vi "TEST - Initialize Array to Path Array.vi"(8 "error in (no error)":errorcluster) -> (0 "error out":errorcluster, 2 "Pass?":bool=TRUE)   [LabVIEW 2009]
doc: "This VI template can be used for the functional testing of VIs; this implementation includes handling for the testing of polymorphic VIs, and the polymorphic elements should be removed if not needed.\n\nCoded by Douglas A. Femec, January 24, 2006.\n\nCopyright (c) 2005-2006 MKS Instruments, Inc.\nAll rights reserved."
uses:
  TEST - Initialize Array from Array - Inputs.ctl
  tests/Polymorphizer+ Data Type.ctl
  TEST - Initialize Array from Array - Outputs.ctl
  Initialize Array from Array/Initialize 1D Array (Path) from 1D Array (EXT).vi
  Initialize Array from Array/Initialize 2D Array (Path) from 2D Array (EXT).vi
  Initialize Array from Array/Initialize 1D Array (Path) from 1D Array (DBL).vi
  Initialize Array from Array/Initialize 2D Array (Path) from 2D Array (DBL).vi
  Initialize Array from Array/Initialize 1D Array (Path) from 1D Array (SGL).vi
  Initialize Array from Array/Initialize 2D Array (Path) from 2D Array (SGL).vi
  Initialize Array from Array/Initialize 1D Array (Path) from 1D Array (I32).vi
  Initialize Array from Array/Initialize 2D Array (Path) from 2D Array (I32).vi
  Initialize Array from Array/Initialize 1D Array (Path) from 1D Array (I64).vi
  Initialize Array from Array/Initialize 2D Array (Path) from 2D Array (I64).vi
  Initialize Array from Array/Initialize 1D Array (Path) from 1D Array (U64).vi
  Initialize Array from Array/Initialize 1D Array (Path) from 1D Array (I16).vi
  Initialize Array from Array/Initialize 2D Array (Path) from 2D Array (I16).vi
  Initialize Array from Array/Initialize 1D Array (Path) from 1D Array (I8).vi
  Initialize Array from Array/Initialize 2D Array (Path) from 2D Array (I8).vi
  Initialize Array from Array/Initialize 1D Array (Path) from 1D Array (U32).vi
  Initialize Array from Array/Initialize 2D Array (Path) from 2D Array (U32).vi
  Initialize Array from Array/Initialize 1D Array (Path) from 1D Array (U16).vi
  Initialize Array from Array/Initialize 2D Array (Path) from 2D Array (U16).vi
  Initialize Array from Array/Initialize 1D Array (Path) from 1D Array (U8).vi
  Initialize Array from Array/Initialize 2D Array (Path) from 2D Array (U8).vi
  Initialize Array from Array/Initialize 1D Array (Path) from 1D Array (Boolean).vi
  Initialize Array from Array/Initialize 2D Array (Path) from 2D Array (Boolean).vi
  Initialize Array from Array/Initialize 1D Array (Path) from 1D Array (String).vi
  Initialize Array from Array/Initialize 2D Array (Path) from 2D Array (String).vi
  Initialize Array from Array/Initialize 1D Array (Path) from 1D Array (Path).vi
  Initialize Array from Array/Initialize 2D Array (Path) from 2D Array (Path).vi
  Initialize Array from Array/Initialize 1D Array (Path) from 1D Array (Variant).vi
  Initialize Array from Array/Initialize 2D Array (Path) from 2D Array (Variant).vi
panel:
  out "Generated Outputs":T1[][](array[typedef]) {"1D Array" format="%.2f"; "2D Array" format="%.2f"}
  in  "Expected Outputs":T1[](array[typedef])=[{"Description"="Expect empty arrays", "1D Array"=[], "2D Array"=[]}, {"Description"="Expect 1-element arrays", "1D Array"=[1.0], "2D Array"=[[1.0]]}, {"Description"="Expect 1-row arrays", "1D Array"=[1.0], "2D Array"=[[1.0, 1.0]]}, {"Description"="Expect 1-column arrays", "1D Array"=[1.0], "2D Array"=[[1.0], [1.0], [1.0], [1.0]]}, {"Description"="Expect 2-columns, 4-rows arrays", "1D Array"=[1.0, 1.0, 1.0, 1.0], "2D Array"=[[1.0, 1.0], [1.0, 1.0], [1.0, 1.0], [1.0, 1.0]]}] {"1D Array" format="%.2f"; "2D Array" format="%.2f"}
  in  "Inputs":T2[](array[typedef])=[{"Description"="Empty arrays", "Data Types to Test"=[enum."EXT", enum."DBL", enum."SGL", enum."I32", enum."I16", enum."I8", enum."U32", enum."U16", enum."U8", enum."Boolean", enum."String", enum."Path", enum."Variant", enum."I64", enum."U64"], "1D Array"=[], "2D Array"=[]}, {"Description"="1-Element arrays", "Data Types to Test"=[enum."EXT", enum."DBL", enum."SGL", enum."I32", enum."I16", enum."I8", enum."U32", enum."U16", enum."U8", enum."Boolean", enum."String", enum."Path", enum."Variant", enum."I64", enum."U64"], "1D Array"=[1.0], "2D Array"=[[1.0]]}, {"Description"="1-Row arrays", "Data Types to Test"=[enum."EXT", enum."DBL", enum."SGL", enum."I32", enum."I16", enum."I8", enum."U32", enum."U16", enum."U8", enum."Boolean", enum."String", enum."Path", enum."Variant", enum."I64", enum."U64"], "1D Array"=[1.0], "2D Array"=[[1.0, 1.0]]}, {"Description"="1-Column arrays", "Data Types to Test"=[enum."EXT", enum."DBL", enum."SGL", enum."I32", enum."I16", enum."I8", enum."U32", enum."U16", enum."U8", enum."Boolean", enum."String", enum."Path", enum."Variant", enum."I64", enum."U64"], "1D Array"=[1.0], "2D Array"=[[1.0], [1.0], [1.0], [1.0]]}, {"Description"="2-Columns, 4-rows arrays", "Data Types to Test"=[enum."EXT", enum."DBL", enum."SGL", enum."I32", enum."I16", enum."I8", enum."U32", enum."U16", enum."U8", enum."Boolean", enum."String", enum."Path", enum."Variant", enum."I64", enum."U64"], "1D Array"=[1.0, 1.0, 1.0, 1.0], "2D Array"=[[1.0, 1.0], [1.0, 1.0], [1.0, 1.0], [1.0, 1.0]]}] {"1D Array" format="%.2f"; "2D Array" format="%.2f"}
  # "Copyright (c) 2005-2006 MKS Instruments, Inc.\nAll rights reserved."
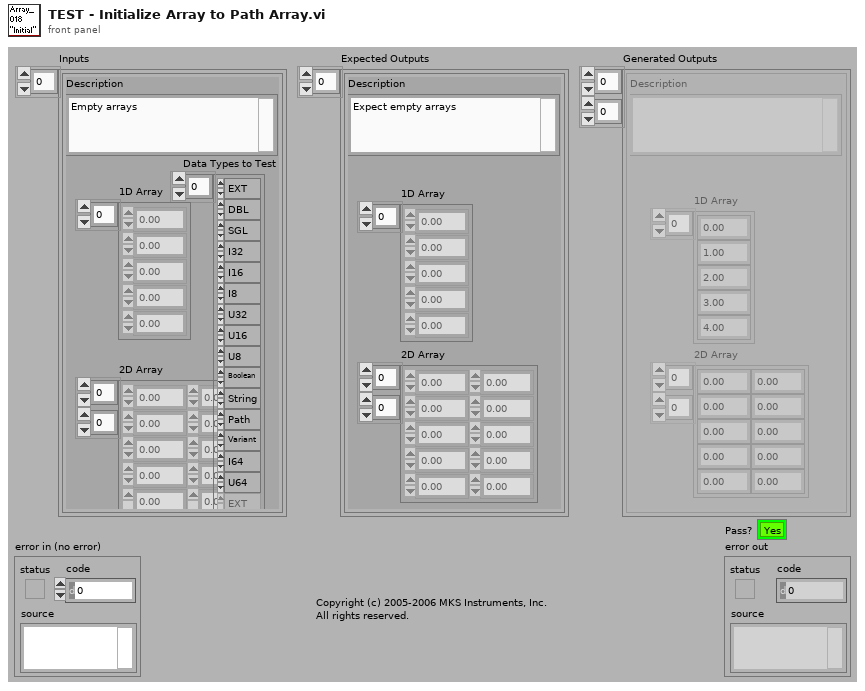
[diagram p1: front panel]
types:
  T1 = typedef "TEST - Initialize Array from Array - Outputs.ctl" = cluster{"Description":string, "1D Array":sgl[], "2D Array":sgl[][]}
  T2 = typedef "TEST - Initialize Array from Array - Inputs.ctl" = cluster{"Description":string, "Data Types to Test":T3[], "1D Array":sgl[], "2D Array":sgl[][]}
  T3 = typedef "Polymorphizer+ Data Type.ctl" = enum16{"EXT", "DBL", "SGL", "I32", "I16", "I8", "U32", "U16", "U8", "CXT", "CDB", "CSG", "Boolean", "String", "Path", "Variant", "CTL-REF", "GEN-REF", "GObj-REF", "VI-REF", "ENUM", "ERR", "FILE-REF", "MENU-REF", "MENU-RING", "PICT-RING", "TXT&PICT-RING", "TXT-RING", "I64", "U64", "LabVIEW Object"}
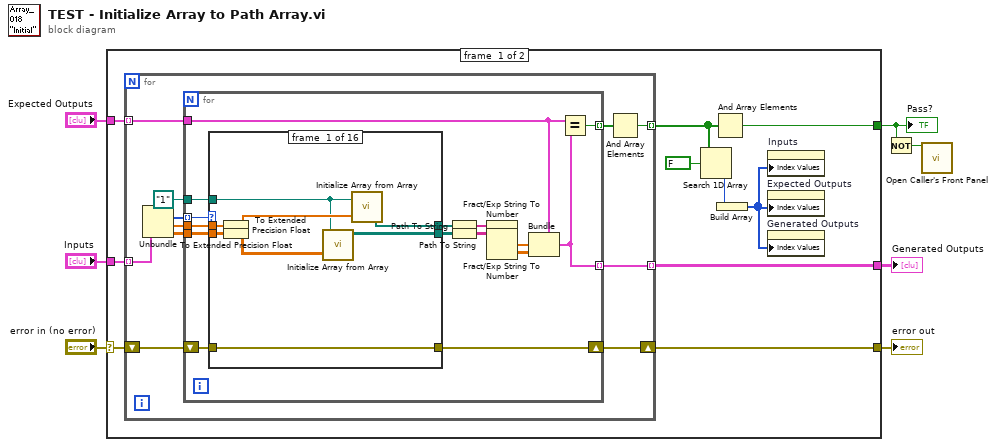
[diagram p0: block diagram]
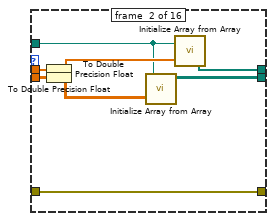
[diagram p2: hidden frame]
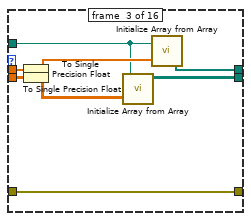
[diagram p3: hidden frame]
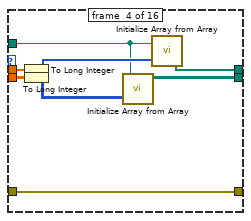
[diagram p4: hidden frame]
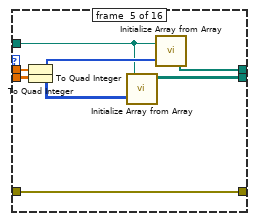
[diagram p5: hidden frame]
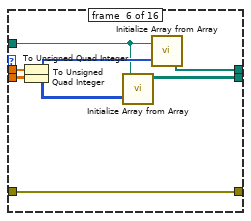
[diagram p6: hidden frame]
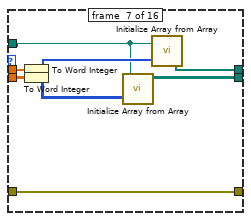
[diagram p7: hidden frame]
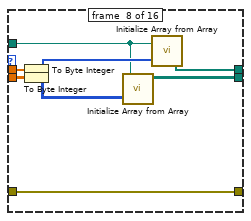
[diagram p8: hidden frame]
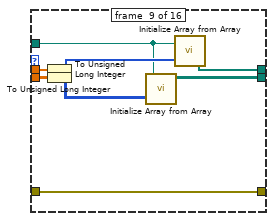
[diagram p9: hidden frame]
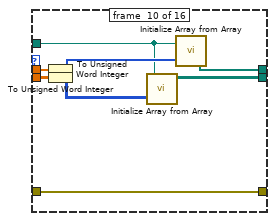
[diagram p10: hidden frame]
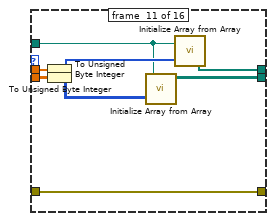
[diagram p11: hidden frame]
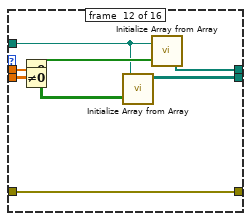
[diagram p12: hidden frame]
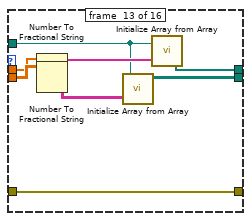
[diagram p13: hidden frame]
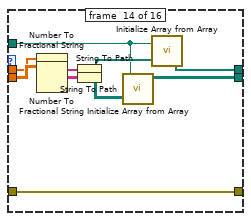
[diagram p14: hidden frame]
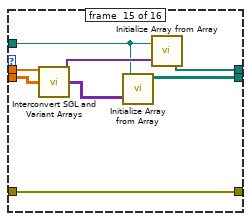
[diagram p15: hidden frame]
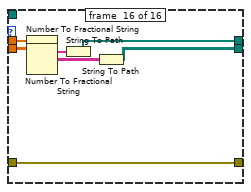
[diagram p16: hidden frame]
diagram:
  n1 = case shown="No Error" "error in (no error)" {
    selector: "error in (no error)" -> [w16 w173]
    tunnel: [w17 w173] -> w6
    tunnel: "Expected Outputs" -> [w14 _]
    tunnel: "Inputs" -> [w15 _]
    tunnel: [w13 _] -> w3
    tunnel: [w12 _] -> w1
    frame #0 {
      n2 = for {
        shift-right: [w23] -> w17
        shift-left: w16 -> [w24]
        tunnel: w15 -> [w25] mode=indexing
        tunnel: w14 -> [w28] mode=indexing
        tunnel: [w27] -> w13 mode=indexing
        tunnel: [w22] -> w11 mode=indexing
        n3 = Unbundle(w25) -> ("Data Types to Test"=w19:T3[], "1D Array"=w20:sgl[], "2D Array"=w21:sgl[][])  [unwired: 1 out]
        n4 = for {
          tunnel: w28 -> [w43]
          tunnel: [w41] -> w27 mode=indexing
          tunnel: [w42] -> w26 mode=indexing
          shift-right: [w36] -> w23
          shift-left: w24 -> [w37]
          tunnel: w19 -> [w38] mode=indexing
          tunnel: w20 -> [w40]
          tunnel: w21 -> [w39]
          tunnel: path "1" -> [w35]
          n5 = case shown="\"U64\"" w38 {
            tunnel: w40 -> [w50 w58 w66 w74 w82 w90 w98 w106 w114 w122 w130 w138 w146 w154 w163 w168]
            tunnel: [w48 w56 w61 w70 w78 w86 w93 w101 w109 w117 w128 w133 w141 w149 w159 w166] -> w31
            tunnel: [w47 w53 w64 w72 w80 w88 w96 w104 w112 w120 w127 w132 w140 w148 w158 w167] -> w32
            tunnel: w39 -> [w51 w59 w67 w75 w83 w91 w99 w107 w115 w123 w131 w139 w147 w156 w164 w169]
            tunnel: w37 -> [w49 w57 w65 w73 w81 w89 w97 w105 w113 w121 w129 w137 w145 w153 w165 w172]
            tunnel: [w49 w57 w65 w73 w81 w89 w97 w105 w113 w121 w129 w137 w145 w153 w165 w172] -> w36
            tunnel: w35 -> [w44 w52 w60 w68 w76 w84 w92 w100 w108 w116 w124 w134 w142 w150 w160 _]
            frame #0 {
              n6 = To Extended Precision Float(1:w50) -> (0:w45:ext[])
              n7 = To Extended Precision Float(1:w51) -> (0:w46:ext[][])
              n8 = call-poly "Initialize Array from Array.vi"("Input Array"=w46, "Element Data"=w44) -> ("Output Array"=w47:path[][])
              n9 = call-poly "Initialize Array from Array.vi"("Input Array"=w45, "Element Data"=w44) -> ("Output Array"=w48:path[])
            }
            frame #1 {
              n10 = To Double Precision Float(number=w58) -> (double precision float=w55:dbl[])
              n11 = To Double Precision Float(number=w59) -> (double precision float=w54:dbl[][])
              n12 = call-poly "Initialize Array from Array.vi"("Input Array"=w54, "Element Data"=w52) -> ("Output Array"=w53:path[][])
              n13 = call-poly "Initialize Array from Array.vi"("Input Array"=w55, "Element Data"=w52) -> ("Output Array"=w56:path[])
            }
            frame #2 {
              n14 = To Single Precision Float(number=w66) -> (single precision float=w63:sgl[])
              n15 = To Single Precision Float(number=w67) -> (single precision float=w62:sgl[][])
              n16 = call-poly "Initialize Array from Array.vi"("Input Array"=w62, "Element Data"=w60) -> ("Output Array"=w64:path[][])
              n17 = call-poly "Initialize Array from Array.vi"("Input Array"=w63, "Element Data"=w60) -> ("Output Array"=w61:path[])
            }
            frame #3 {
              n18 = To Long Integer(number=w74) -> (32bit integer=w69:i32[])
              n19 = To Long Integer(number=w75) -> (32bit integer=w71:i32[][])
              n20 = call-poly "Initialize Array from Array.vi"("Input Array"=w71, "Element Data"=w68) -> ("Output Array"=w72:path[][])
              n21 = call-poly "Initialize Array from Array.vi"("Input Array"=w69, "Element Data"=w68) -> ("Output Array"=w70:path[])
            }
            frame #4 {
              n22 = To Quad Integer(1:w82) -> (0:w77:i64[])
              n23 = To Quad Integer(1:w83) -> (0:w79:i64[][])
              n24 = call-poly "Initialize Array from Array.vi"("Input Array"=w79, "Element Data"=w76) -> ("Output Array"=w80:path[][])
              n25 = call-poly "Initialize Array from Array.vi"("Input Array"=w77, "Element Data"=w76) -> ("Output Array"=w78:path[])
            }
            frame #5 {
              n26 = To Unsigned Quad Integer(1:w90) -> (0:w85:u64[])
              n27 = To Unsigned Quad Integer(1:w91) -> (0:w87:u64[][])
              n28 = call-poly "Initialize Array from Array.vi"("Input Array"=w87, "Element Data"=w84) -> ("Output Array"=w88:path[][])
              n29 = call-poly "Initialize Array from Array.vi"("Input Array"=w85, "Element Data"=w84) -> ("Output Array"=w86:path[])
            }
            frame #6 {
              n30 = To Word Integer(number=w98) -> (16bit integer=w95:i16[])
              n31 = To Word Integer(number=w99) -> (16bit integer=w94:i16[][])
              n32 = call-poly "Initialize Array from Array.vi"("Input Array"=w94, "Element Data"=w92) -> ("Output Array"=w96:path[][])
              n33 = call-poly "Initialize Array from Array.vi"("Input Array"=w95, "Element Data"=w92) -> ("Output Array"=w93:path[])
            }
            frame #7 {
              n34 = To Byte Integer(number=w106) -> (8bit integer=w103:i8[])
              n35 = To Byte Integer(number=w107) -> (8bit integer=w102:i8[][])
              n36 = call-poly "Initialize Array from Array.vi"("Input Array"=w102, "Element Data"=w100) -> ("Output Array"=w104:path[][])
              n37 = call-poly "Initialize Array from Array.vi"("Input Array"=w103, "Element Data"=w100) -> ("Output Array"=w101:path[])
            }
            frame #8 {
              n38 = To Unsigned Long Integer(number=w114) -> (unsigned 32bit integer=w111:u32[])
              n39 = To Unsigned Long Integer(number=w115) -> (unsigned 32bit integer=w110:u32[][])
              n40 = call-poly "Initialize Array from Array.vi"("Input Array"=w110, "Element Data"=w108) -> ("Output Array"=w112:path[][])
              n41 = call-poly "Initialize Array from Array.vi"("Input Array"=w111, "Element Data"=w108) -> ("Output Array"=w109:path[])
            }
            frame #9 {
              n42 = To Unsigned Word Integer(number=w122) -> (unsigned 16bit integer=w119:u16[])
              n43 = To Unsigned Word Integer(number=w123) -> (unsigned 16bit integer=w118:u16[][])
              n44 = call-poly "Initialize Array from Array.vi"("Input Array"=w118, "Element Data"=w116) -> ("Output Array"=w120:path[][])
              n45 = call-poly "Initialize Array from Array.vi"("Input Array"=w119, "Element Data"=w116) -> ("Output Array"=w117:path[])
            }
            frame #10 {
              n46 = To Unsigned Byte Integer(number=w130) -> (unsigned 8bit integer=w125:u8[])
              n47 = To Unsigned Byte Integer(number=w131) -> (unsigned 8bit integer=w126:u8[][])
              n48 = call-poly "Initialize Array from Array.vi"("Input Array"=w126, "Element Data"=w124) -> ("Output Array"=w127:path[][])
              n49 = call-poly "Initialize Array from Array.vi"("Input Array"=w125, "Element Data"=w124) -> ("Output Array"=w128:path[])
            }
            frame #11 {
              n50 = Not Equal To 0?(x=w138) -> (x != 0?=w136:bool[])
              n51 = Not Equal To 0?(x=w139) -> (x != 0?=w135:bool[][])
              n52 = call-poly "Initialize Array from Array.vi"("Input Array"=w135, "Element Data"=w134) -> ("Output Array"=w132:path[][])
              n53 = call-poly "Initialize Array from Array.vi"("Input Array"=w136, "Element Data"=w134) -> ("Output Array"=w133:path[])
            }
            frame #12 {
              n54 = Number To Fractional String(number=w146) -> (F-format string=w144:string[])  [unwired: 3 in]
              n55 = Number To Fractional String(number=w147) -> (F-format string=w143:string[][])  [unwired: 3 in]
              n56 = call-poly "Initialize Array from Array.vi"("Input Array"=w143, "Element Data"=w142) -> ("Output Array"=w140:path[][])
              n57 = call-poly "Initialize Array from Array.vi"("Input Array"=w144, "Element Data"=w142) -> ("Output Array"=w141:path[])
            }
            frame #13 {
              n58 = Number To Fractional String(number=w154) -> (F-format string=w155:string[])  [unwired: 3 in]
              n59 = Number To Fractional String(number=w156) -> (F-format string=w157:string[][])  [unwired: 3 in]
              n60 = String To Path(string=w155) -> (path=w152:path[])
              n61 = String To Path(string=w157) -> (path=w151:path[][])
              n62 = call-poly "Initialize Array from Array.vi"("Input Array"=w151, "Element Data"=w150) -> ("Output Array"=w148:path[][])
              n63 = call-poly "Initialize Array from Array.vi"("Input Array"=w152, "Element Data"=w150) -> ("Output Array"=w149:path[])
            }
            frame #14 {
              n64 = call "Interconvert SGL and Variant Arrays.vi"("SGL 1D Array In"=w163, "SGL 2D Array In"=w164) -> ("Variant 1D Array Out"=w162:variant[], "Variant 2D Array Out"=w161:variant[][])  [unwired: 9 in, 3 out]
              n65 = call-poly "Initialize Array from Array.vi"("Input Array"=w161, "Element Data"=w160) -> ("Output Array"=w158:path[][])
              n66 = call-poly "Initialize Array from Array.vi"("Input Array"=w162, "Element Data"=w160) -> ("Output Array"=w159:path[])
            }
            frame #15 {
              n67 = Number To Fractional String(number=w168) -> (F-format string=w170:string[])  [unwired: 3 in]
              n68 = Number To Fractional String(number=w169) -> (F-format string=w171:string[][])  [unwired: 3 in]
              n69 = String To Path(string=w170) -> (path=w166:path[])
              n70 = String To Path(string=w171) -> (path=w167:path[][])
            }
          }
          n71 = Path To String(path=w31) -> (string=w29:string[])
          n72 = Path To String(path=w32) -> (string=w30:string[][])
          n73 = Fract/Exp String To Number(string=w29) -> (number=w33:dbl[])  [unwired: 3 in, 1 out]
          n74 = Fract/Exp String To Number(string=w30) -> (number=w34:dbl[][])  [unwired: 3 in, 1 out]
          n75 = Bundle(cluster=w43, "1D Array"=w33, "2D Array"=w34) -> (w41:T1)  [unwired: 1 in]
          n76 = Equal?(x=w43, y=w41) -> (x = y?=w42:bool)
        }
        n77 = And Array Elements(Boolean array=w26) -> (logical AND=w22:bool)
      }
      n78 = Search 1D Array(1D array=w11, element=FALSE) -> (index of element=w9:i32)  [unwired: 1 in]
      n79 = And Array Elements(Boolean array=w11) -> (logical AND=w12:bool)
      n80 = Build Array(w9) -> (w8:i32[])
      n81 = property on="Inputs" class="Arr (strict)"("Index Values"=w8) -> ()  [unwired: 2 in, 2 out]
      n82 = property on="Expected Outputs" class="Arr (strict)"("Index Values"=w8) -> ()  [unwired: 2 in, 2 out]
      n83 = property on="Generated Outputs" class="Arr (strict)"("Index Values"=w8) -> ()  [unwired: 2 in, 2 out]
    }
    frame #1 {
    }
  }
  "error out" <- w6
  "Pass?" <- w1
  "Generated Outputs" <- w3
  n84 = Not(x=w1) -> (.not. x?=w2:bool)
  n85 = call "Open Caller's Front Panel.vi"("Open?"=w2) -> ()  [unwired: 14 in, 1 out]
